vi "Check if Process if Running.vi"(8 "error in (no error)":errorcluster, 10 "Process Name":string) -> (0 "error out":errorcluster, 2 "Running?":bool)   [LabVIEW 2014, in "NIPM_API.lvlib"]
uses:
  NIPM_API.lvlib
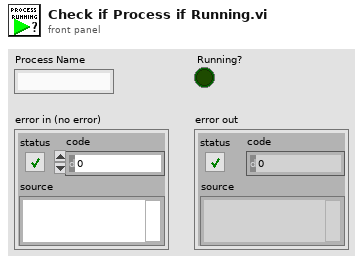
[diagram p1: front panel]
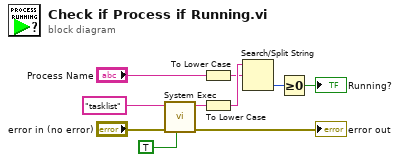
[diagram p0: block diagram]
diagram:
  n1 = call <vilib>:"System Exec.vi"("run minimized? (F)"=TRUE, "error in (no error)"="error in (no error)", "command line"="tasklist") -> ("error out"=→"error out":errorcluster, "standard output"=w6:string)  [unwired: 5 in, 2 out]
  n2 = To Lower Case(string="Process Name") -> (all lower case string=w3:string)
  n3 = To Lower Case(string=w6) -> (all lower case string=w5:string)
  n4 = Search/Split String(string=w5, search string/char (-)=w3) -> (offset of match=w2:i32)  [unwired: 1 in, 2 out]
  n5 = Greater Or Equal To 0?(x=w2) -> (x >= 0?=→"Running?":bool)
